vi "SLAM_Calc.vi"() -> ()   [LabVIEW 2015]
panel:
  in  "Straightened":bool=TRUE
  out "XY Graph":cluster{i32[], i32[]}[](graph)
  in  "Robot Input":bool
  out "error out":errorcluster
  in  "error in (no error)":errorcluster
  in  "Bluetooth Port":refnum<visa-resource-name>
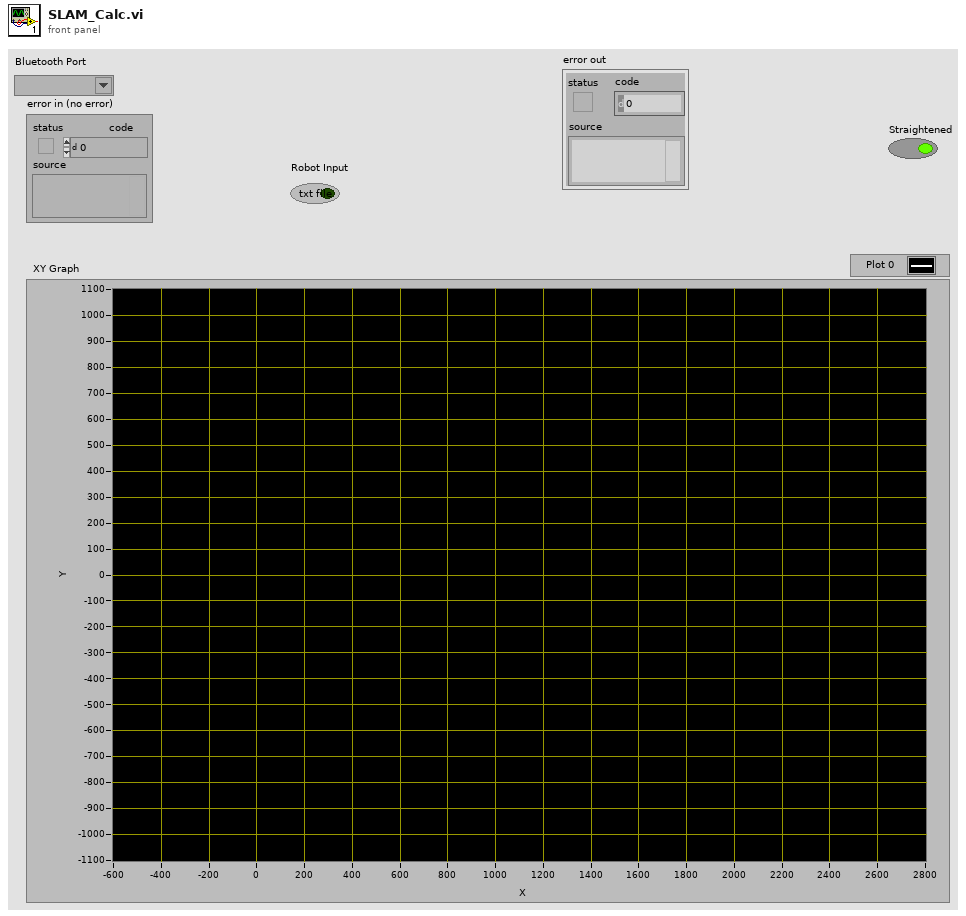
[diagram p1: front panel]
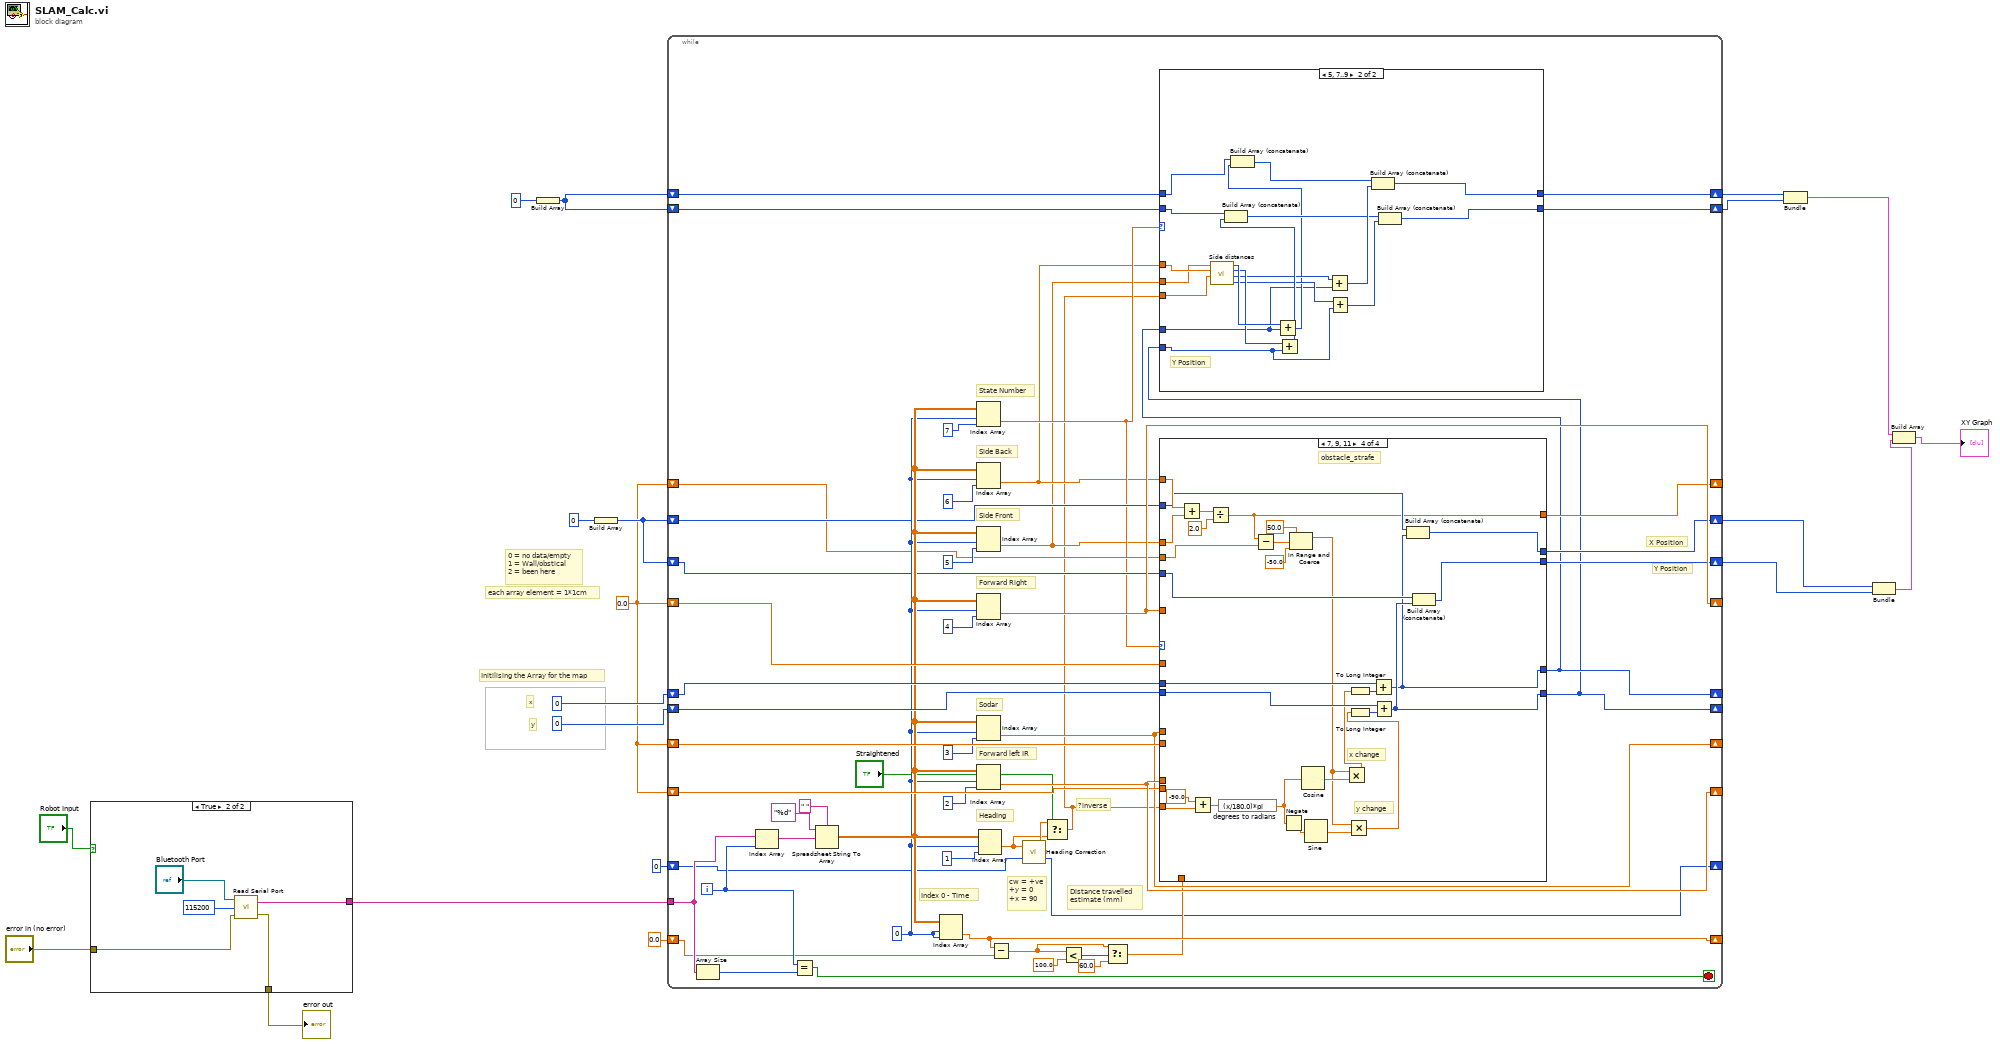
[diagram p0: block diagram]
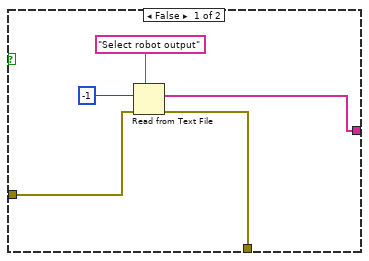
[diagram p2: hidden frame]
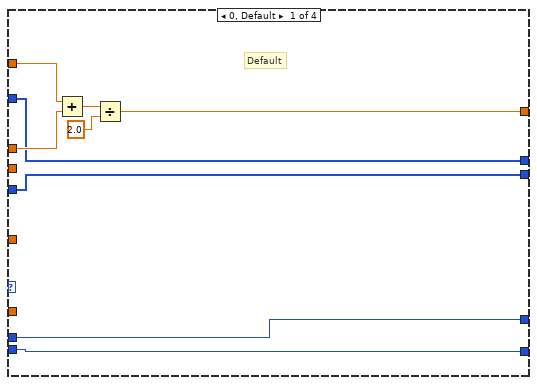
[diagram p4: hidden frame]
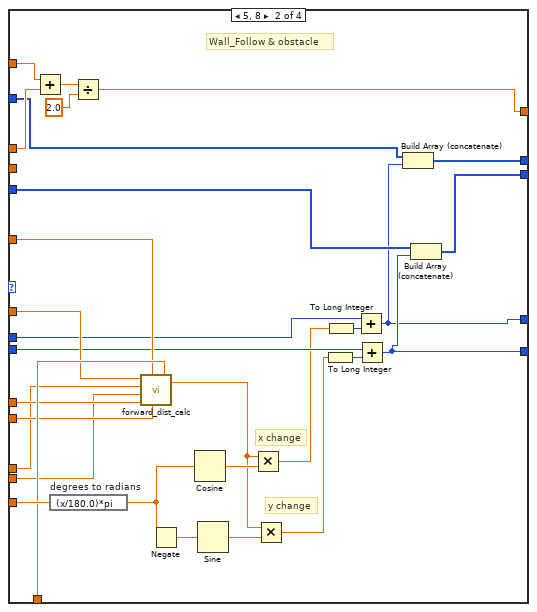
[diagram p5: hidden frame]
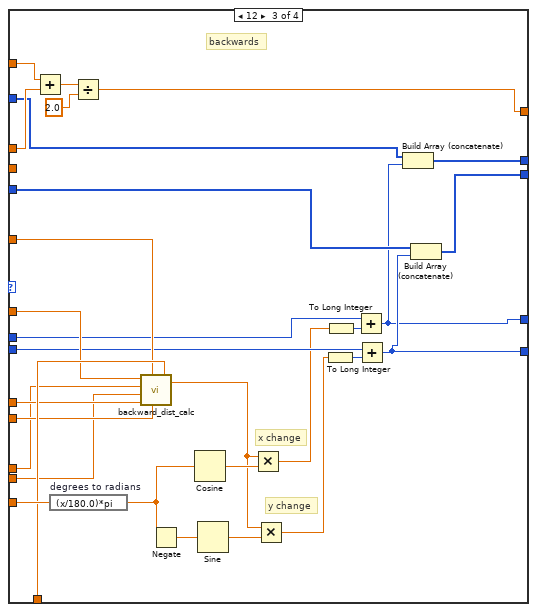
[diagram p6: hidden frame]
diagram:
  w9 = 0.0 ("element")
  # "y"
  # "x"
  # "each array element = 1*1cm"
  # "0 = no data/empty\n1 = Wall/obstical\n2 = been here"
  # "Initilising the Array for the map"
  n1 = case shown="True" "Robot Input" {
    tunnel: [w21 w28] -> w20
    tunnel: "error in (no error)" -> [w24 w27]
    tunnel: [w23 w26] -> w17
    frame False {
      n2 = Read from Text File(prompt (Open existing file)="Select robot output", count=-1, error in=w24) -> (text=w21:string[], error out=w23:errorcluster)  [unwired: 1 in, 2 out]
    }
    frame True {
      n3 = call "Read Serial Port.vi"("error in (no error)"=w27, "baud rate"=u32 115200, "Bluetooth Port"="Bluetooth Port") -> ("error out"=w26:errorcluster, "Output Data"=w28:string[])
    }
  }
  "error out" <- w17
  n4 = Build Array(0) -> (w7:i32[])
  n5 = Build Array(0) -> (w12:i32[])
  n6 = while {
    tunnel: w20 -> [w81]
    shift-right: [w40] -> _
    shift-left: 0 ("index (row)") -> [w76]
    shift-right: [w39] -> _
    shift-left: 0 ("disabled index (col)") -> [w75]
    shift-right: [w73] -> _
    shift-left: w9 -> [w68]
    shift-right: [w66] -> _
    shift-left: w9 -> [w70]
    shift-right: [w74] -> _
    shift-left: w9 -> [w69]
    shift-right: [w72] -> _
    shift-left: 0.0 ("element") -> [w71]
    shift-right: [w67] -> _
    shift-left: w9 -> [w48]
    shift-right: [w46] -> w11
    shift-left: w12 -> [w54]
    shift-right: [w45] -> w10
    shift-left: w12 -> [w55]
    shift-right: [w37] -> w5
    shift-left: w7 -> [w41]
    shift-right: [w38] -> w6
    shift-left: w7 -> [w42]
    shift-right: [w36] -> _
    shift-left: 0 ("Count Out") -> [w35]
    i -> [w80]
    stop <- w82 stop-if-true
    w56 = 0 ("index (row)")
    # "Y Position"
    # "X Position"
    # "?inverse"
    # "cw = +ve\n+y = 0\n+x = 90"
    # "State Number"
    # "Side Back"
    # "Side Front"
    # "Forward Right"
    # "Sodar"
    # "Forward left IR"
    # "Heading"
    # "Distance travelled \nestimate (mm)"
    # "Index 0 - Time"
    n7 = Array Size(array=w81) -> (size(s)=w79:i32)
    n8 = Index Array(array=w81, index=w80) -> (element=w78:string)
    n9 = Equal?(x=w80, y=w79) -> (x = y?=w82:bool)
    n10 = Spreadsheet String To Array(delimiter (Tab)=" ", format string="%d", spreadsheet string=w78) -> (array=w58:dbl[][])  [unwired: 1 in]
    n11 = Index Array(array=w58, index (row)=w56, index (col)=w56) -> (element=w72:dbl)
    n12 = Index Array(array=w58, index (row)=w56, index (col)=7 ("index (row)")) -> (element=w47:dbl)
    n13 = Index Array(array=w58, index (row)=w56, index (col)=6 ("index (row)")) -> (element=w44:dbl)
    n14 = Index Array(array=w58, index (row)=w56, index (col)=5 ("index (row)")) -> (element=w43:dbl)
    n15 = Index Array(array=w58, index (row)=w56, index (col)=4 ("index (row)")) -> (element=w73:dbl)
    n16 = Index Array(array=w58, index (row)=w56, index (col)=3 ("index (row)")) -> (element=w66:dbl)
    n17 = Index Array(array=w58, index (row)=w56, index (col)=2 ("index (row)")) -> (element=w74:dbl)
    n18 = Index Array(array=w58, index (row)=w56, index (col)=1 ("disabled index (col)")) -> (element=w32:dbl)
    n19 = Subtract(x=w72, y=w71) -> (x-y=w51:dbl)
    n20 = call "Heading Correction.vi"("Count In"=w35, "Current Heading"=w32) -> ("Count Out"=w36:i32, "Transformed Heading"=w33:dbl)
    n21 = Select(t=w33, s="Straightened", f=w32) -> (s? t:f=w34:dbl)
    n22 = Less?(x=w51, y=100.0) -> (x < y?=w52:bool)
    n23 = Select(t=w51, s=w52, f=60.0) -> (s? t:f=w49:dbl)
    n24 = case shown="7, 9, 11" w47 {
      tunnel: w74 -> [_ w138 w168 _]
      tunnel: w66 -> [_ w140 w170 _]
      tunnel: w73 -> [_ w135 w165 _]
      tunnel: w43 -> [w107 w121 w151 w200]
      tunnel: w44 -> [w108 w122 w152 w201]
      tunnel: w34 -> [_ w142 w172 w191]
      tunnel: w76 -> [w111 w130 w160 w196]
      tunnel: w75 -> [w112 w129 w159 w195]
      tunnel: [w111 w116 w146 w179] -> w40
      tunnel: [w112 w117 w147 w180] -> w39
      tunnel: w49 -> [_ w141 w171 _]
      tunnel: w70 -> [_ w139 w169 _]
      tunnel: w69 -> [_ w137 w167 _]
      tunnel: w68 -> [_ w136 w166 _]
      tunnel: [w106 w120 w150 w182] -> w67
      tunnel: w55 -> [w105 w119 w149 w185]
      tunnel: [w105 w118 w148 w183] -> w45
      tunnel: w54 -> [w104 w115 w145 w186]
      tunnel: [w104 w114 w144 w184] -> w46
      tunnel: w48 -> [_ _ _ w181]
      frame 0, Default {
        # "Default"
        n25 = Add(x=w108, y=w107) -> (x+y=w110:dbl)
        n26 = Divide(x=w110, y=2.0) -> (x/y=w106:dbl)
      }
      frame 5, 8 {
        # "y change"
        # "x change"
        # "Wall_Follow & obstacle"
        n27 = Add(x=w122, y=w121) -> (x+y=w124:dbl)
        n28 = expression code="(x/180.0)*pi" "degrees to radians"(w142) -> (w134:dbl)
        n29 = Divide(x=w124, y=2.0) -> (x/y=w120:dbl)
        n30 = call "forward_dist_calc.vi"("dt"=w141, "Sodar Past"=w139, "Forward Right"=w135, "Sodar"=w140, "Forward Left Past"=w137, "Forward Left"=w138, "Forward Right Past"=w136) -> ("Forward distance"=w131:dbl)
        n31 = Negate(x=w134) -> (-x=w113:dbl)
        n32 = Cosine(x=w134) -> (cos(x)=w133:dbl)
        n33 = Sine(x=w113) -> (sin(x)=w132:dbl)
        n34 = Multiply(x=w131, y=w133) -> (x*y=w127:dbl)
        n35 = Multiply(x=w131, y=w132) -> (x*y=w128:dbl)
        n36 = To Long Integer(number=w128) -> (32bit integer=w126:i32)
        n37 = To Long Integer(number=w127) -> (32bit integer=w125:i32)
        n38 = Add(x=w130, y=w125) -> (x+y=w116:i32)
        n39 = Add(x=w129, y=w126) -> (x+y=w117:i32)
        n40 = Build Array (concatenate)(w115, w116) -> (w114:i32[])
        n41 = Build Array (concatenate)(w119, w117) -> (w118:i32[])
      }
      frame 12 {
        # "y change"
        # "x change"
        # "backwards"
        n42 = Add(x=w152, y=w151) -> (x+y=w154:dbl)
        n43 = expression code="(x/180.0)*pi" "degrees to radians"(w172) -> (w164:dbl)
        n44 = Divide(x=w154, y=2.0) -> (x/y=w150:dbl)
        n45 = call "backward_dist_calc.vi"("dt"=w171, "Sodar Past"=w169, "Forward Right"=w165, "Sodar"=w170, "Forward Left Past"=w167, "Forward Left"=w168, "Forward Right Past"=w166) -> ("Forward distance"=w161:dbl)
        n46 = Negate(x=w164) -> (-x=w143:dbl)
        n47 = Cosine(x=w164) -> (cos(x)=w163:dbl)
        n48 = Sine(x=w143) -> (sin(x)=w162:dbl)
        n49 = Multiply(x=w161, y=w163) -> (x*y=w157:dbl)
        n50 = Multiply(x=w161, y=w162) -> (x*y=w158:dbl)
        n51 = To Long Integer(number=w158) -> (32bit integer=w156:i32)
        n52 = To Long Integer(number=w157) -> (32bit integer=w155:i32)
        n53 = Add(x=w160, y=w155) -> (x+y=w146:i32)
        n54 = Add(x=w159, y=w156) -> (x+y=w147:i32)
        n55 = Build Array (concatenate)(w145, w146) -> (w144:i32[])
        n56 = Build Array (concatenate)(w149, w147) -> (w148:i32[])
      }
      frame 7, 9, 11 {
        # "y change"
        # "x change"
        # "obstacle_strafe"
        n57 = Add(x=w201, y=w200) -> (x+y=w199:dbl)
        n58 = Add(x=-90.0, y=w191) -> (x+y=w192:dbl)
        n59 = Divide(x=w199, y=2.0) -> (x/y=w182:dbl)
        n60 = expression code="(x/180.0)*pi" "degrees to radians"(w192) -> (w174:dbl)
        n61 = Subtract(x=w182, y=w181) -> (x-y=w178:dbl)
        n62 = Negate(x=w174) -> (-x=w173:dbl)
        n63 = In Range and Coerce(upper limit=50.0, x=w178, lower limit=-50.0) -> (coerced(x)=w177:dbl)  [unwired: 1 out]
        n64 = Cosine(x=w174) -> (cos(x)=w193:dbl)
        n65 = Sine(x=w173) -> (sin(x)=w194:dbl)
        n66 = Multiply(x=w177, y=w193) -> (x*y=w188:dbl)
        n67 = Multiply(x=w177, y=w194) -> (x*y=w189:dbl)
        n68 = To Long Integer(number=w188) -> (32bit integer=w187:i32)
        n69 = To Long Integer(number=w189) -> (32bit integer=w197:i32)
        n70 = Add(x=w196, y=w187) -> (x+y=w179:i32)
        n71 = Add(x=w195, y=w197) -> (x+y=w180:i32)
        n72 = Build Array (concatenate)(w186, w179) -> (w184:i32[])
        n73 = Build Array (concatenate)(w185, w180) -> (w183:i32[])
      }
    }
    n74 = case shown="5, 7..9" w47 {
      tunnel: w40 -> [_ w86]
      tunnel: w39 -> [_ w85]
      tunnel: w44 -> [_ w101]
      tunnel: w43 -> [_ w100]
      tunnel: w42 -> [w84 w89]
      tunnel: w41 -> [w83 w102]
      tunnel: w34 -> [_ w99]
      tunnel: [w83 w91] -> w37
      tunnel: [w84 w90] -> w38
      frame 0, Default {
      }
      frame 5, 7..9 {
        # "Y Position"
        n75 = call "Side distances.vi"("Heading"=w99, "side back"=w101, "side front"=w100) -> (0:"side front y"=w95:i32, "side back x"=w96:i32, 2:"side front y"=w97:i32, "side front x"=w98:i32)  [unwired: 1 in]
        n76 = Add(x=w98, y=w86) -> (x+y=w88:i32)
        n77 = Build Array (concatenate)(w89, w88) -> (w87:i32[])
        n78 = Add(x=w97, y=w85) -> (x+y=w103:i32)
        n79 = Build Array (concatenate)(w102, w103) -> (w93:i32[])
        n80 = Add(x=w96, y=w86) -> (x+y=w94:i32)
        n81 = Add(x=w95, y=w85) -> (x+y=w92:i32)
        n82 = Build Array (concatenate)(w87, w94) -> (w90:i32[])
        n83 = Build Array (concatenate)(w93, w92) -> (w91:i32[])
      }
    }
  }
  n84 = Bundle(w6, w5) -> (w4:cluster{i32[], i32[]})  [unwired: 1 in]
  n85 = Bundle(w11, w10) -> (w3:cluster{i32[], i32[]})  [unwired: 1 in]
  n86 = Build Array(w4, w3) -> (→"XY Graph":cluster{i32[], i32[]}[])
